vi "Config-Meas-Timing.vi"(6 "# PLCs for long integration time":i32=16, 7 "short integration time\n(rounded to the nearest multiple of 80us)":dbl=0.00064 format="%^.0e", 8 "error in (no error)":errorcluster, 9 "wait time parameter":dbl=1.0 format="%.1f", 10 "integration time":i32(slide) scale=0.0..2.0, 11 "VISA session":refnum<visa-resource-name>) -> (0 "error out":errorcluster, 3 "VISA resource name out":refnum<visa-resource-name>)   [LabVIEW 2016]
doc: "This VI configures the timing parameters of the measurement functions. The settings of this VI could be different from the actual instrument's settings due to limits imposed by other parameters inside the instrument. To check the actual values of integration time and number of power line cycles, run HP415xA Query Integration Time.vi."
panel:
  # "(wait time = wait time parameter * default wait time)"
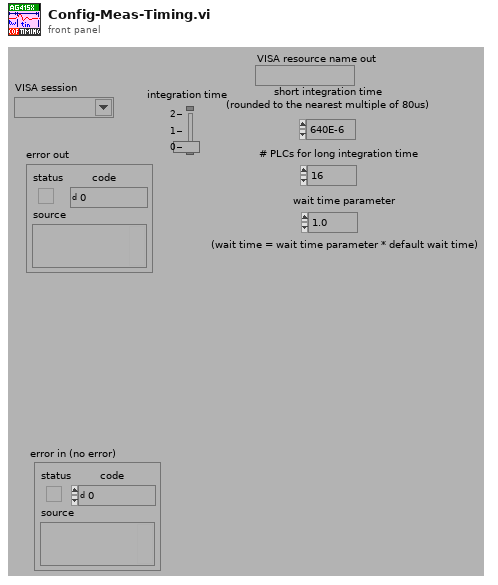
[diagram p1: front panel]
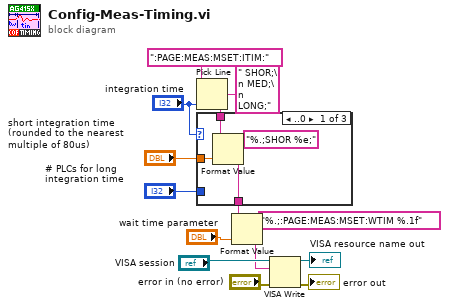
[diagram p0: block diagram]
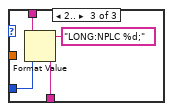
[diagram p3: hidden frame]
diagram:
  n1 = Pick Line(string ("")=":PAGE:MEAS:MSET:ITIM:", multi-line string=" SHOR;\n MED;\n LONG;", line index="integration time") -> (output string=w10:string)
  n2 = case shown="..0" "integration time" {
    tunnel: w10 -> [w18 w19 w23]
    tunnel: "# PLCs for long integration time" -> [_ _ w20]
    tunnel: "short integration time\n(rounded to the nearest multiple of 80us)" -> [w17 _ _]
    tunnel: [w15 w19 w21] -> w5
    frame ..0 {
      n3 = Format Value(string ("")=w18, format string="%.;SHOR %e;", value (0)=w17) -> (output string=w15:string)
    }
    frame 1 {
    }
    frame 2.. {
      n4 = Format Value(string ("")=w23, format string="LONG:NPLC %d;", value (0)=w20) -> (output string=w21:string)
    }
  }
  n5 = Format Value(string ("")=w5, format string="%.;:PAGE:MEAS:MSET:WTIM %.1f", value (0)="wait time parameter") -> (output string=w3:string)
  n6 = VISA Write(VISA resource name="VISA session", write buffer=w3, error in (no error)="error in (no error)") -> (VISA resource name out=→"VISA resource name out":refnum<visa-resource-name>, error out=→"error out":errorcluster)  [unwired: 1 out]
